vi "EditarOnda.vi"(7 "LabVIEW Web Service Request":refnum<class "Web Request.lvclass">, 9 "Cursor1":dbl, 10 "Cursor0":dbl, 11 "Edicao":i32) -> ()   [LabVIEW 2020]
uses:
  <vilib>/wsapi/Web Request.lvclass
  5af7745c-4718-4284-8f9d-5e540539c5d7.vi
panel:
  # "Use the Web Service Request input terminal to call the VIs on the Web Services palette. Do not remove it from the connector pane unless you don't need access to the palette."
  # "Each additional control wired to the connector pane will be available as an input in the URL. To include an indicator in terminal-mode output (the default setting), it must also be wired to the connector pane."
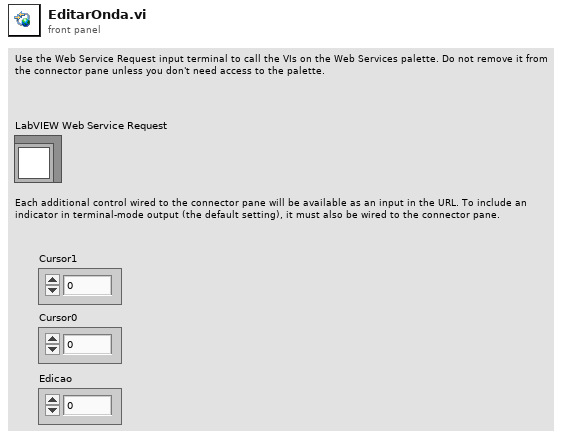
[diagram p1: front panel]
types:
  T1 = enum16{"create", "fire - Simular onda", "fire - Editar onda", "destroy"}
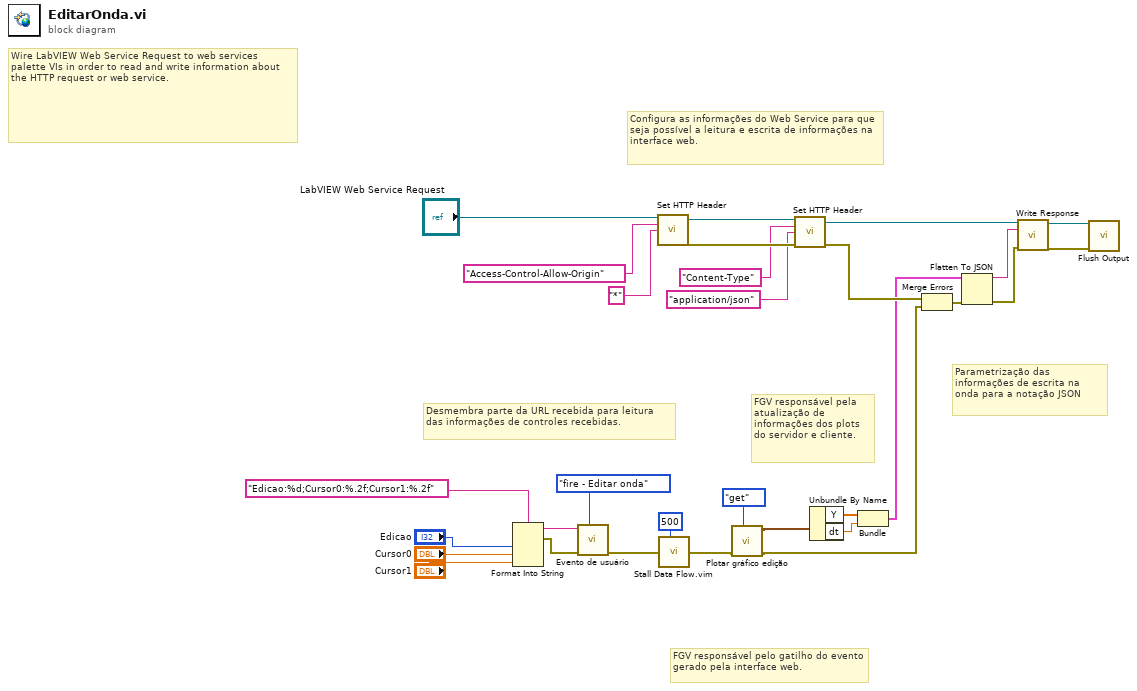
[diagram p0: block diagram]
diagram:
  # "Parametrização das informações de escrita na onda para a notação JSON"
  # "FGV responsável pela atualização de informações dos plots do servidor e cliente."
  # "FGV responsável pelo gatilho do evento gerado pela interface web."
  # "Desmembra parte da URL recebida para leitura das informações de controles recebidas."
  # "Configura as informações do Web Service para que seja possível a leitura e escrita de informações na interface web."
  # "Wire LabVIEW Web Service Request to web services palette VIs in order to read and write information about the HTTP request or web service."
  n1 = Format Into String(format string="Edicao:%d;Cursor0:%.2f;Cursor1:%.2f", "Edicao", "Cursor0", "Cursor1") -> (resulting string=w19:string, error out=w17:errorcluster)  [unwired: 2 in]
  n2 = call "Evento de usuário.vi"("Enum"=T1."fire - Editar onda", "error in (no error)"=w17, "Dados"=w19) -> ("error out"=w18:errorcluster)  [unwired: 7 in, 1 out]
  n3 = call <vilib>:"Set HTTP Header.vi"("LabVIEW Web Service Request"="LabVIEW Web Service Request", "header"="Access-Control-Allow-Origin", "header value"="*") -> ("LabVIEW Web Service Request out"=w30:refnum<class "Web Request.lvclass">, "error out"=w29:errorcluster)  [unwired: 11 in]
  n4 = call "Stall Data Flow.vim"("value in"=w18, "milliseconds to wait"=u32 500) -> ("value out"=w9:errorcluster)  [unwired: 1 out]
  n5 = call "Plotar gráfico edição.vi"("Enum"=enum16{"set", "get"}."get", "error in (no error)"=w9) -> ("error out"=w8:errorcluster, "Plot"=w7:waveform(dbl))  [unwired: 8 in]
  n6 = call <vilib>:"Set HTTP Header.vi"("LabVIEW Web Service Request"=w30, "header"="Content-Type", "header value"="application/json", "error in (no error)"=w29) -> ("LabVIEW Web Service Request out"=w28:refnum<class "Web Request.lvclass">, "error out"=w16:errorcluster)  [unwired: 10 in]
  n7 = Unbundle By Name(w7) -> ("Y"=w15:dbl[], "dt"=w14:dbl)
  n8 = Bundle("Y"=w15, "dt"=w14) -> (w13:cluster{"Y":dbl[], "dt":dbl})  [unwired: 1 in]
  n9 = Merge Errors(w16, w8) -> (w11:errorcluster)
  n10 = Flatten To JSON(anything=w13, error in (no error)=w11) -> (JSON string=w21:string, 11:w1:errorcluster)  [unwired: 1 in]
  n11 = call <vilib>:"Write Response.vi"("LabVIEW Web Service Request"=w28, "response string"=w21, "error in (no error)"=w1) -> ("LabVIEW Web Service Request out"=w23:refnum<class "Web Request.lvclass">, "error out"=w22:errorcluster)  [unwired: 11 in]
  n12 = call <vilib>:"Flush Output.vi"("LabVIEW Web Service Request"=w23, "error in (no error)"=w22) -> ()  [unwired: 12 in, 2 out]
